vi "Write StationOptions.vi"(8 "error in (no error)":errorcluster, 10 "StationOptions":T8={"DataBase"={"Connection String Expression"="", "User ID"="", "Password"=""}, "Local Report"={"Report Path"=path "", "Report  Format"=enum."CSV", "Disabled State"=FALSE, "Customer name"=""}, "Localization"={"Language"=enum."English"}, "Preferences"={"Station ID"="", "IP Address"="", "Password"=""}, "  User Manager"={"Current User Manager File"="", "Login on start"=FALSE}, "Multiple UUT Settings"={"Number of Tests Sockets"=1, "Synchronization"=enum."Don't Synchronize"}, "Sequence"={"Sequence Folder Path"=path ""}} {"Multiple UUT Settings"."Number of Tests Sockets" min=1 step=1}, 11 "StationOptions in":refnum<class "StationOptions.lvclass">) -> (0 "error out":errorcluster, 3 "StationOptions out":refnum<class "StationOptions.lvclass">)   [LabVIEW 2019, in "SoftwareSetup.lvlib" / "StationOptions.lvclass"]
uses:
  StationOptions.lvclass
  DataBase.ctl
  Local Report.ctl
  Localization.ctl
  Preferences.ctl
  User Manager.ctl
  Multiple UUT Settings.ctl
  Sequence.ctl
  StationOptions.lvclass/StationOptions.ctl
  SoftwareSetup.lvlib
panel:
  # "Number of Tests Sockets"
  # "Synchronization"
  # "User Manager File"
  # "Station Info"
  # "MES Info"
  # "Select a Language:"
  # "Report File"
  # "Data Link Options"
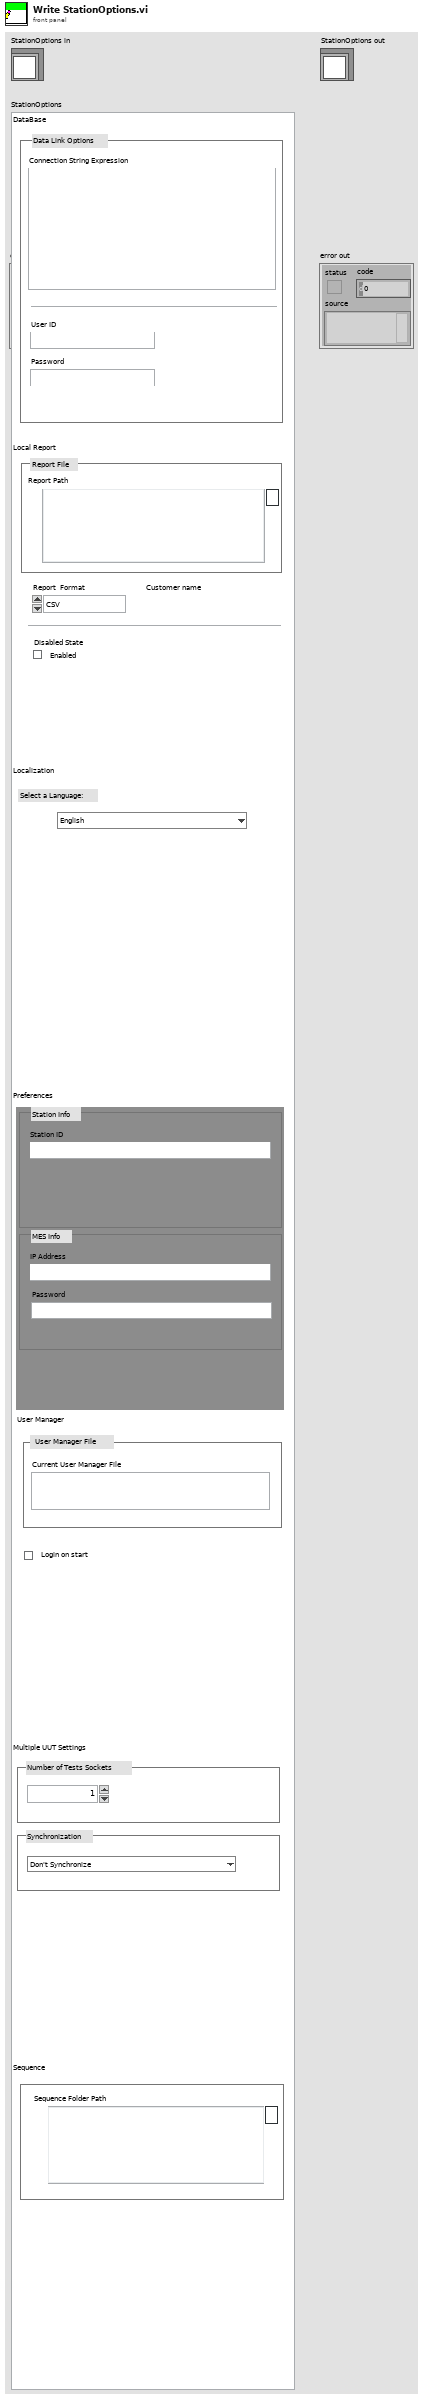
[diagram p1: front panel]
types:
  T1 = typedef "SoftwareSetup.lvlib/DataBase.ctl" = cluster{"Connection String Expression":string, "User ID":string, "Password":string}
  T2 = typedef "SoftwareSetup.lvlib/Local Report.ctl" = cluster{"Report Path":path, "Report  Format":enum16{"CSV", "XML", "PDF", "Excel", "TXT"}, "Disabled State":bool, "Customer name":string}
  T3 = typedef "SoftwareSetup.lvlib/Localization.ctl" = cluster{"Language":enum16{"English", "Chinese"}}
  T4 = typedef "SoftwareSetup.lvlib/Preferences.ctl" = cluster{"Station ID":string, "IP Address":string, "Password":string}
  T5 = typedef "SoftwareSetup.lvlib/User Manager.ctl" = cluster{"Current User Manager File":string, "Login on start":bool}
  T6 = typedef "SoftwareSetup.lvlib/Multiple UUT Settings.ctl" = cluster{"Number of Tests Sockets":u8, "Synchronization":enum16{"Don't Synchronize", "Serial", "Parallel", "One Thread Only"}}
  T7 = typedef "SoftwareSetup.lvlib/Sequence.ctl" = cluster{"Sequence Folder Path":path}
  T8 = cluster{"DataBase":T1, "Local Report":T2, "Localization":T3, "Preferences":T4, "  User Manager":T5, "Multiple UUT Settings":T6, "Sequence":T7}
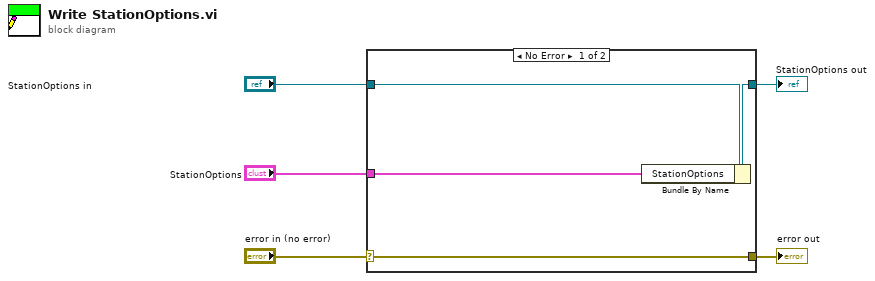
[diagram p0: block diagram]
diagram:
  n1 = case shown="No Error" "error in (no error)" {
    selector: "error in (no error)" -> [w9 w10]
    tunnel: [w9 w10] -> w4
    tunnel: [w7 w11] -> w2
    tunnel: "StationOptions in" -> [w8 w11]
    tunnel: "StationOptions" -> [w6 _]
    frame No Error {
      n2 = Bundle By Name(cluster=w8, "StationOptions"=w6) -> (w7:refnum<class "StationOptions.lvclass">)
    }
    frame Error {
    }
  }
  "error out" <- w4
  "StationOptions out" <- w2
